vi "Separate IP from Port.vi"(10 "IP+Port":string) -> (1 "Port":u16, 2 "IP":string)   [LabVIEW 2026]
uses:
  Global Constants.vi
  TALOS.lvlib
panel:
  out "Textual Port":string
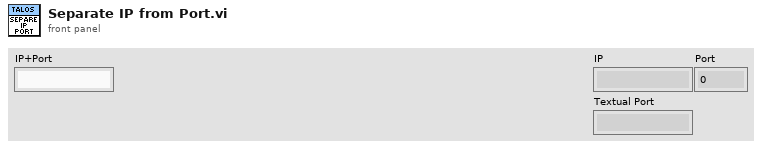
[diagram p1: front panel]
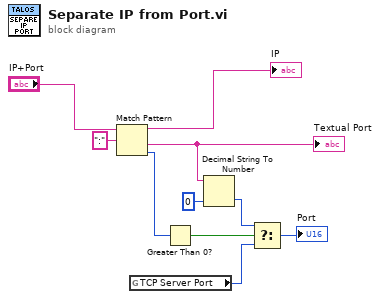
[diagram p0: block diagram]
diagram:
  n1 = Match Pattern(string="IP+Port", regular expression=":") -> (before substring=→"IP":string, after substring=w4:string, offset past match=w7:i32)  [unwired: 1 in, 1 out]
  "Textual Port" <- w4
  n2 = global read "Global Constants.vi" "TCP Server Port"() -> (w5:u16)
  n3 = Greater Than 0?(x=w7) -> (x > 0?=w6:bool)
  n4 = Decimal String To Number(string=w4, default (0L)=u16 0 ("default (0 I32)")) -> (number=w2:u16)  [unwired: 1 in, 1 out]
  n5 = Select(t=w2, s=w6, f=w5) -> (s? t:f=→"Port":u16)
